vi "WriteInputFilter.vi"(11 "Controller Sampling Frequency [Hz]":dbl=50000.0 format="%#_13g") -> (2 "K_filt_sos_den":dbl[](array[numeric]), 3 "K_filt_sos_num":dbl[](array[numeric]))   [LabVIEW 2016]
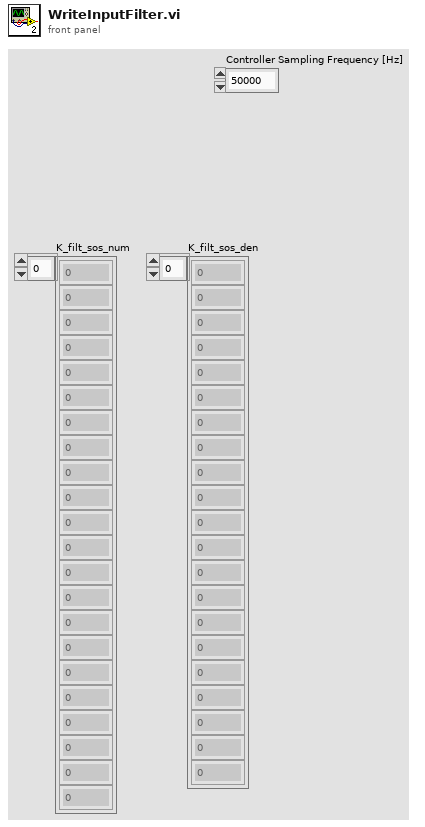
[diagram p1: front panel]
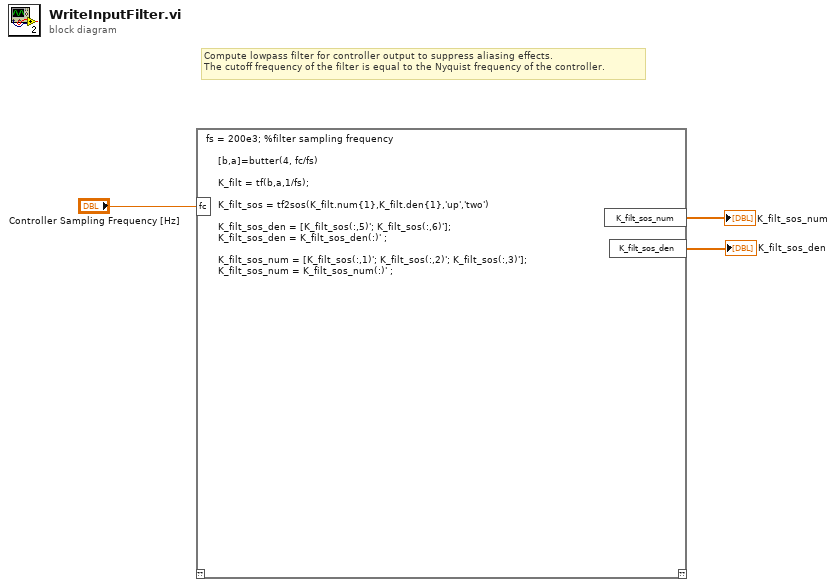
[diagram p0: block diagram]
diagram:
  # "Compute lowpass filter for controller output to suppress aliasing effects.\nThe cutoff frequency of the filter is equal to the Nyquist frequency of the controller."
  n1 = script code="fs = 200e3; %filter sampling frequency\n\n    [b,a]=butter(4, fc/fs)\n\n    K_filt = tf(b,a,1/fs);\n\n    K_filt_sos = tf2sos(K_filt.num{1},K_filt.den{1},'up','two')\n\n    K_filt_sos_den = [K_filt_sos(:,5)'; K_filt_sos(:,6)'];\n    K_filt_sos_den = K_filt_sos_den(:)' ; \n\n    K_filt_sos_num = [K_filt_sos(:,1)'; K_filt_sos(:,2)'; K_filt_sos(:,3)'];\n    K_filt_sos_num = K_filt_sos_num(:)' ;"("fc"="Controller Sampling Frequency [Hz]") -> ("K_filt_sos_num"=→"K_filt_sos_num":dbl[], "K_filt_sos_den"=→"K_filt_sos_den":dbl[])  [unwired: 1 in, 1 out]
